vi "Has Permission.vi"(11 "Session Data":refnum<class "Session.lvclass">) -> (3 "Has Permission":bool)   [LabVIEW 2026, in "Session.lvclass"]
uses:
  Session.lvclass
  Session.lvclass/Session.ctl
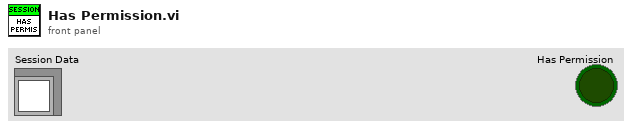
[diagram p1: front panel]
types:
  T1 = typedef "Role Enum.ctl" = enum16{"Operator", "Engineer", "Admin"}
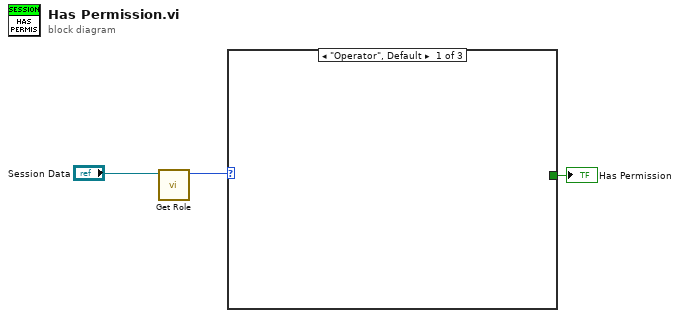
[diagram p0: block diagram]
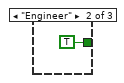
[diagram p2: hidden frame]
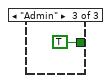
[diagram p3: hidden frame]
diagram:
  n1 = call "Get Role.vi"("Session Data"="Session Data") -> ("Role"=w2:T1)  [unwired: 10 in]
  n2 = case shown="\"Operator\", Default" w2 {
    tunnel: [_ TRUE TRUE] -> w1
    frame "Operator", Default {
    }
    frame "Engineer" {
    }
    frame "Admin" {
    }
  }
  "Has Permission" <- w1
